vi "jettl Msg Teardown.vi"() -> (2 "Msg Strategy":refnum<class "Msg Strategy.lvclass">)   [LabVIEW 2021, in "jettl Msg Teardown.lvlib"]
uses:
  jettl Msg Teardown.lvlib
  jettl/Msg Strategy/Msg Strategy.lvclass
  Teardown Msg Strategy/Teardown Msg Strategy.lvclass
  C:/git/jettl/src/jettl/Msg Strategy/Msg Strategy.lvclass
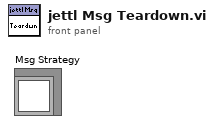
[diagram p1: front panel]
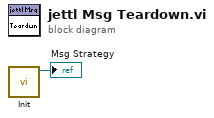
[diagram p0: block diagram]
diagram:
  n1 = call "Init.vi"() -> ("Teardown Msg Strategy out"=→"Msg Strategy":refnum<class "Teardown Msg Strategy.lvclass">)  [unwired: 11 in]
